vi "UMM_LogIn.vi"(8 "error in (no error)":errorcluster caption="错误输入（无错误）", 11 "User Management Model 输入":refnum<class "User Management Model.lvclass">) -> (0 "error out":errorcluster caption="错误输出", 2 "登录信息":T1, 3 "User Management Model 输出":refnum<class "User Management Model.lvclass">)   [LabVIEW 2019, in "User Management Model.lvclass"]
uses:
  User Management Model.lvclass
  protect/ObjectAttributes.ctl
panel:
  in  "取消":bool
  in  "登陆":bool=TRUE
  in  "登出":bool
  in  "管理员登陆":bool
  in  "密码:":string caption="String"
  in  "登录名:":string(combo) caption="Combo Box"
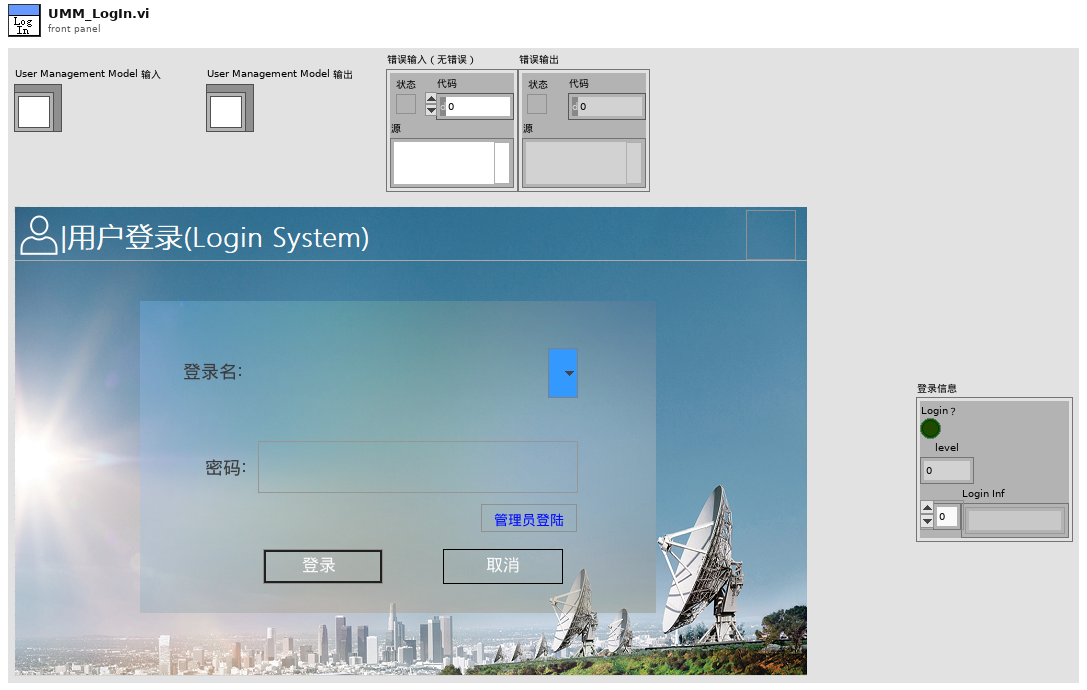
[diagram p1: front panel]
types:
  T1 = typedef "User Management Model.lvclass/ObjectAttributes.ctl" = cluster{"Login？":bool, "level":i32, "Login Inf":string[]}
  T2 = enum16{"open", "replace", "create", "open or create", "replace or create", "replace or create with confirmation"}
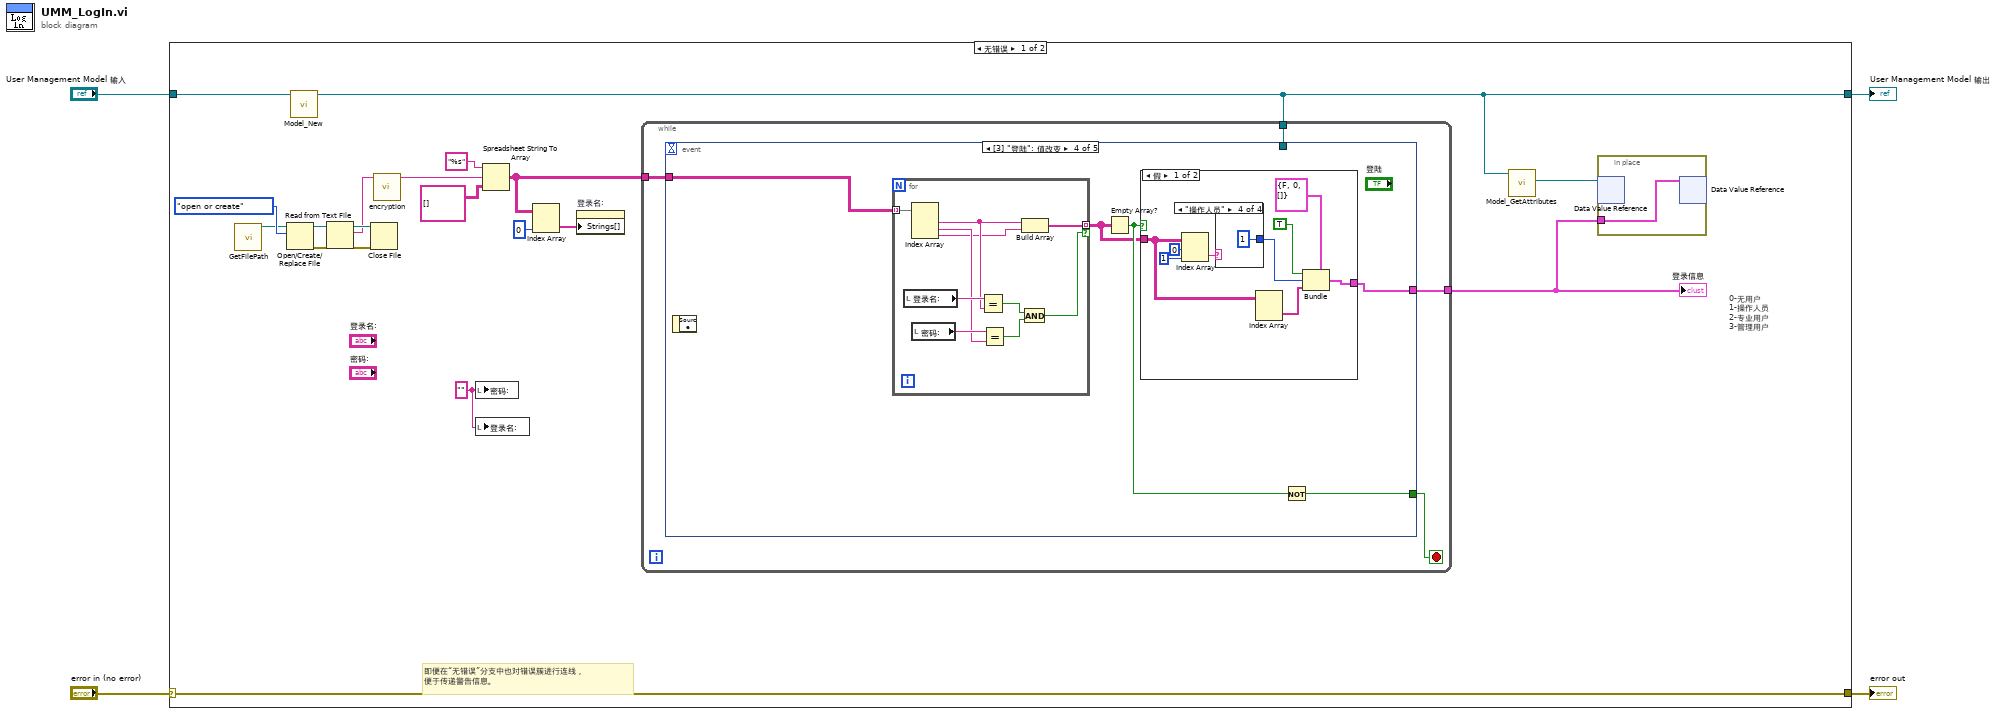
[diagram p0: block diagram]
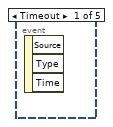
[diagram p2: hidden frame]
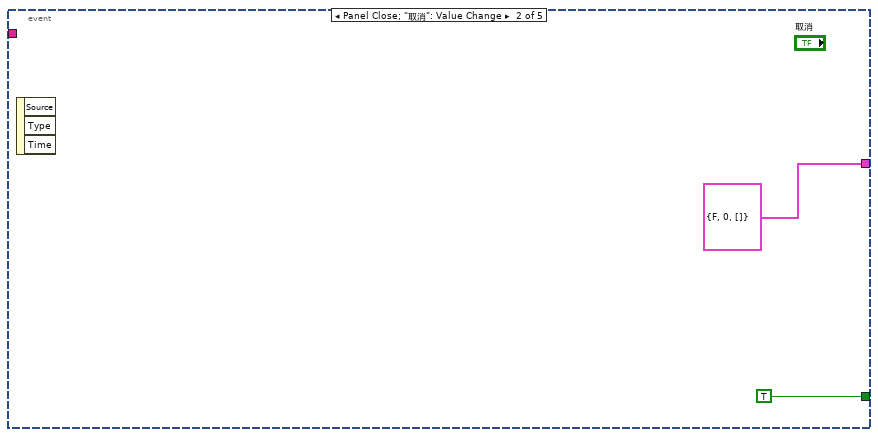
[diagram p3: hidden frame]
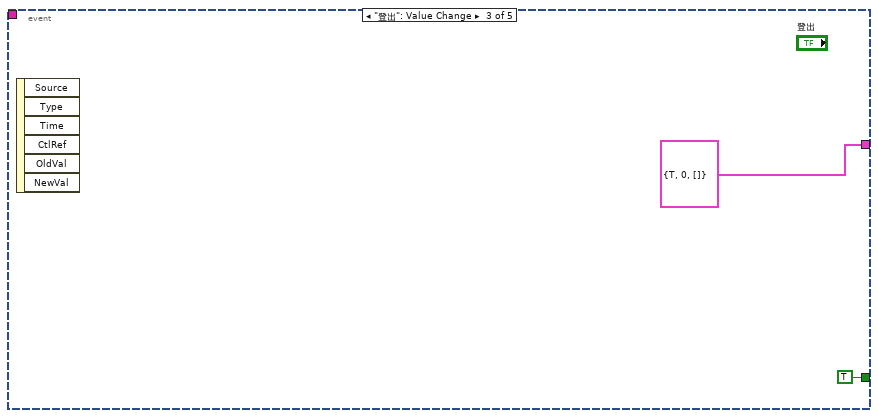
[diagram p4: hidden frame]
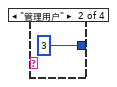
[diagram p6: hidden frame]
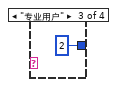
[diagram p7: hidden frame]
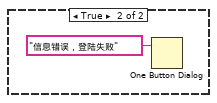
[diagram p8: hidden frame]
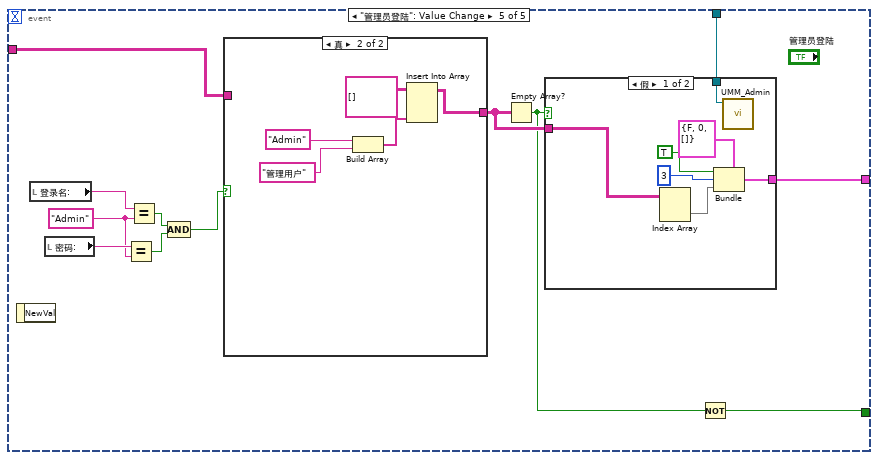
[diagram p9: hidden frame]
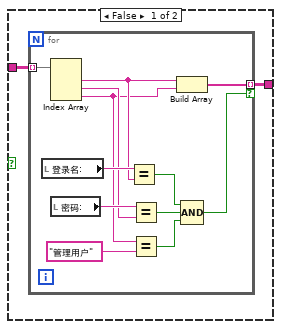
[diagram p10: hidden frame]
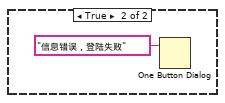
[diagram p11: hidden frame]
diagram:
  n1 = case shown="无错误" "error in (no error)" {
    selector: "error in (no error)" -> [w23 w101]
    tunnel: [w23 w101] -> w3
    tunnel: [w7 w100] -> w1
    tunnel: "User Management Model 输入" -> [w8 w100]
    frame No Error {
      w9 = "" ("密码:")
      # "0-无用户\n1-操作人员\n2-专业用户\n3-管理用户"
      # "即便在“无错误”分支中也对错误簇进行连线，\n便于传递警告信息。"
      n2 = call "GetFilePath.vi"() -> ("添加的路径"=w17:path)  [unwired: 19 in]
      n3 = Open/Create/Replace File(file path (use dialog)=w17, operation (0:open)=T2."open or create" ("操作(0:open)")) -> (refnum out=w21:refnum<file>, error out=w20:errorcluster)  [unwired: 4 in, 1 out]
      n4 = call "Model_New.vi"("User Management Model 输入"=w8) -> ("User Management Model 输出"=w7:refnum<class "User Management Model.lvclass">)  [unwired: 9 in, 1 out]
      n5 = Read from Text File(file (use dialog)=w21, error in=w20) -> (refnum out=w19:refnum<file>, text=w16:string, error out=w18:errorcluster)  [unwired: 2 in, 1 out]
      n6 = Close File(refnum=w19, error in=w18) -> ()  [unwired: 2 out]
      n7 = call "encryption.vi"("字符串"=w16) -> ("转换值"=w15:string)  [unwired: 10 in]
      n8 = local write "密码:"(w9) -> ()
      n9 = local write "登录名:"(w9) -> ()
      n10 = Spreadsheet String To Array(format string="%s" ("格式字符串"), spreadsheet string=w15, array type (2D Dbl)=string[][] [] ("格式字符串")) -> (array=w12:string[][])  [unwired: 1 in]
      n11 = Index Array(array=w12, index (col)=0 ("禁用的索引 (列)")) -> (element=w10:string[])  [unwired: 1 in]
      n12 = property on="登录名:" class="CmbBox"("Strings[]"=w10) -> ()  [unwired: 2 in, 2 out]
      n13 = while {
        tunnel: w12 -> [w28]
        tunnel: [w25] -> w5
        tunnel: w7 -> [w26]
        stop <- w27 stop-if-true
        n14 = event shown="[3] \"登陆\": 值改变" {
          selector: _ -> [_ _ _ _ _]
          dyn-events: _ -> [_ _ _ _ _]
          timeout: _ -> [_ _ _ _ _]
          tunnel: w28 -> [_ _ _ w37 w71]
          tunnel: [_ TRUE TRUE w36 w69] -> w27
          tunnel: w26 -> [_ _ _ _ w62]
          tunnel: [_ T1 {"Login？"=FALSE, "level"=0, "Login Inf"=[]} ("登录信息") T1 {"Login？"=TRUE, "level"=0, "Login Inf"=[]} ("登录信息") w33 w61] -> w25
          event Timeout {
            n15 = event-data() -> ()  [unwired: 1 in, 3 out]
          }
          event Panel Close; "取消": Value Change {
            n16 = event-data() -> ()  [unwired: 1 in, 3 out]
          }
          event "登出": Value Change {
            n17 = event-data() -> ()  [unwired: 1 in, 6 out]
          }
          event "登陆": Value Change {
            n18 = event-data() -> ()  [unwired: 1 in, 1 out]
            n19 = for {
              tunnel: w37 -> [w60] mode=indexing
              tunnel: [w54] -> w34 mode=indexing if=w51
              n20 = local read "登录名:"() -> (w59:string)
              n21 = Index Array(array=w60) -> (element #1=w56:string, element #2=w57:string, element #3=w55:string)  [unwired: 3 in]
              n22 = local read "密码:"() -> (w58:string)
              n23 = Equal?(x=w59, y=w56) -> (x = y?=w53:bool)
              n24 = Equal?(x=w58, y=w57) -> (x = y?=w52:bool)
              n25 = Build Array(w56, w55) -> (w54:string[])
              n26 = Compound Arithmetic op=AND ("复合运算")(w53, w52) -> (w51:bool)
            }
            n27 = Empty Array?(array=w34) -> (empty?=w35:bool)
            n28 = case shown="假" w35 {
              tunnel: w34 -> [w44 _]
              tunnel: [w45 _] -> w33
              frame False {
                n29 = Index Array(array=w44, index (row)=0 ("禁用的索引 (行)"), index (col)=1 ("禁用的索引 (列)")) -> (element=w41:string)
                n30 = case shown="\"操作人员\"" w41 {
                  tunnel: [_ 3 2 1] -> w40
                  frame Default {
                  }
                  frame "管理用户" {
                  }
                  frame "专业用户" {
                  }
                  frame "操作人员" {
                  }
                }
                n31 = Index Array(array=w44) -> (element=w46:string[])  [unwired: 2 in]
                n32 = Bundle(cluster=T1 {"Login？"=FALSE, "level"=0, "Login Inf"=[]} ("登录信息"), "Login？"=TRUE, "level"=w40, "Login Inf"=w46) -> (w45:T1)
              }
              frame True {
                n33 = One Button Dialog(message="信息错误，登陆失败" ("消息")) -> ()  [unwired: 1 in, 1 out]
              }
            }
            n34 = Not(x=w35) -> (.not. x?=w36:bool)
          }
          event "管理员登陆": Value Change {
            w66 = "Admin" ("y")
            n35 = event-data() -> ()  [unwired: 1 in, 1 out]
            n36 = local read "登录名:"() -> (w68:string)
            n37 = local read "密码:"() -> (w67:string)
            n38 = Equal?(x=w67, y=w66) -> (x = y?=w64:bool)
            n39 = Equal?(x=w68, y=w66) -> (x = y?=w65:bool)
            n40 = Compound Arithmetic op=AND ("复合运算")(w65, w64) -> (w63:bool)
            n41 = case shown="真" w63 {
              tunnel: [w74 w90] -> w72
              tunnel: w71 -> [w73 _]
              frame False {
                n42 = for {
                  tunnel: w73 -> [w86] mode=indexing
                  tunnel: [w81] -> w74 mode=indexing if=w78
                  n43 = local read "登录名:"() -> (w85:string)
                  n44 = Index Array(array=w86) -> (element #1=w82:string, element #2=w83:string, element #3=w77:string)  [unwired: 3 in]
                  n45 = local read "密码:"() -> (w84:string)
                  n46 = Equal?(x=w85, y=w82) -> (x = y?=w80:bool)
                  n47 = Equal?(x=w84, y=w83) -> (x = y?=w79:bool)
                  n48 = Equal?(x=w77, y="管理用户") -> (x = y?=w75:bool)
                  n49 = Build Array(w82, w77) -> (w81:string[])
                  n50 = Compound Arithmetic op=AND ("复合运算")(w80, w79, w75) -> (w78:bool)
                }
              }
              frame True {
                n51 = Build Array("Admin" ("y"), "管理用户" ("元素")) -> (w89:string[])
                n52 = Insert Into Array(array=string[][] [] ("数组"), new element=w89) -> (w90:string[][])  [unwired: 2 in]
              }
            }
            n53 = Empty Array?(array=w72) -> (empty?=w70:bool)
            n54 = case shown="假" w70 {
              tunnel: w72 -> [w98 _]
              tunnel: [w96 _] -> w61
              tunnel: w62 -> [w95 _]
              frame False {
                n55 = Index Array(array=w98) -> (element=w97:string[])  [unwired: 2 in]
                n56 = Bundle(cluster=T1 {"Login？"=FALSE, "level"=0, "Login Inf"=[]} ("登录信息"), "Login？"=TRUE, "level"=3, "Login Inf"=w97) -> (w96:T1)
                n57 = call-dynamic "UMM_Admin.vi"("User Management Model 输入"=w95) -> ()  [unwired: 8 in, 3 out]
              }
              frame True {
                n58 = One Button Dialog(message="信息错误，登陆失败" ("消息")) -> ()  [unwired: 1 in, 1 out]
              }
            }
            n59 = Not(x=w70) -> (.not. x?=w69:bool)
          }
        }
      }
      "登录信息" <- w5
      n60 = call "Model_GetAttributes.vi"("User Management Model 输入"=w7) -> ("属性引用"=w6:refnum<data-value>)  [unwired: 7 in, 3 out]
      n61 = in-place {
        in-place-border: w5 -> [w24]
        n62 = in-place-dvr #1(w6) -> ()  [unwired: 2 out]
        n63 = in-place-dvr #1(w24) -> ()  [unwired: 2 out]
      }
    }
    frame Error {
    }
  }
  "error out" <- w3
  "User Management Model 输出" <- w1
